vi "DeleteTopicConnection.vi"(1 "ROS":T1={"topic port"=0, "Node"="", "topic"="", "type"="", "node port"=0, "error "={"status"=FALSE, "code"=0, "source"=""}, "Direction"=enum."Node", "APIs"=[], "Update (ms)"=1, "write queue"=1}, 2 "Con In":T1[](array[typedef])) -> (0 "Con out":T1[](array[typedef]))   [LabVIEW 2012]
uses:
  <userlib>/ROSforLV/ROS/Code/SubVIs/_ROSControl.ctl
  <userlib>/ROSforLV/ROS/Code/SubVIs/_ROSDirection.ctl
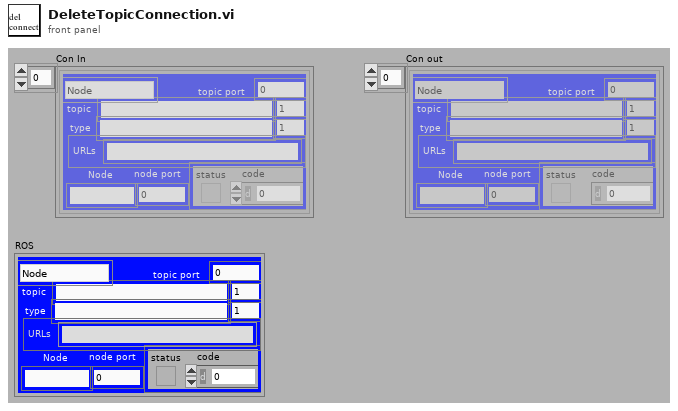
[diagram p1: front panel]
types:
  T1 = typedef "_ROSControl.ctl" = cluster{"topic port":u16, "Node":string, "topic":string, "type":string, "node port":u32, "error ":errorcluster, "Direction":T2, "APIs":string[], "Update (ms)":u16, "write queue":u16}
  T2 = typedef "_ROSDirection.ctl" = enum16{"Node", "Publisher", "Subscriber", "Service Client"}
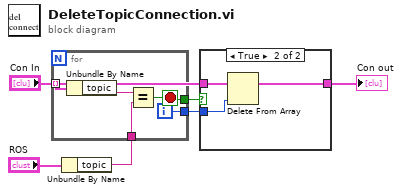
[diagram p0: block diagram]
diagram:
  n1 = Unbundle By Name("ROS") -> ("topic"=w5:string)
  n2 = for {
    tunnel: "Con In" -> [w11] mode=indexing
    tunnel: w5 -> [w9]
    tunnel: [w8] -> w1
    tunnel: [w7] -> w6
    i -> [w8]
    stop <- w7 stop-if-true
    n3 = Unbundle By Name(w11) -> ("topic"=w10:string)
    n4 = Equal?(x=w10, y=w9) -> (x = y?=w7:bool)
  }
  n5 = case shown="True" w6 {
    tunnel: [w12 w15] -> w2
    tunnel: "Con In" -> [w12 w14]
    tunnel: w1 -> [_ w13]
    frame False {
    }
    frame True {
      n6 = Delete From Array(array=w14, index=w13) -> (array with subset deleted=w15:T1[])  [unwired: 1 in, 1 out]
    }
  }
  "Con out" <- w2
